vi "WriteMultipleMessages.vi"(6 "Timeout(ms)":i32, 8 "error in (no error)":errorcluster, 10 "Messages":T1[](array[typedef]), 11 "NetworkConnection in":refnum<class "NetworkConnection.lvclass">) -> (0 "error out":errorcluster, 2 "StillConnected?":bool, 3 "NetworkConnection out":refnum<class "NetworkConnection.lvclass">, 4 "Timed Out?":bool)   [LabVIEW 2020, in "NetworkConnection.lvclass"]
doc: "Writes an array of messages for the Remote System.\n\nJKI Network Streams Connection 1.1.1.15\nJavier Ruiz - JKI\nCopyright (c) 2020, JKI\n\nThis library is provided \"AS IS\" ,WITHOUT WARRANTIES OR CONDITIONS OF ANY KIND, either express or implied."
uses:
  NetworkConnection.lvclass
  NetworkCommand--Cluster.ctl
  NetworkMessage--Cluster.ctl
  NetworkConnection.lvclass/NetworkConnection.ctl
  Clear Errors.vi
  <resource>/objmgr/ni.dex.rc
panel:
  # "Copyright © 2020 JKI All rights reserved.\n\nAuthor: Javier Ruiz <javier.ruiz@jki.net>\n\nThis library is provided \"AS IS\" ,WITHOUT WARRANTIES OR \nCONDITIONS OF ANY KIND, either expressed or implied.\n\nJKI -- jki.net"
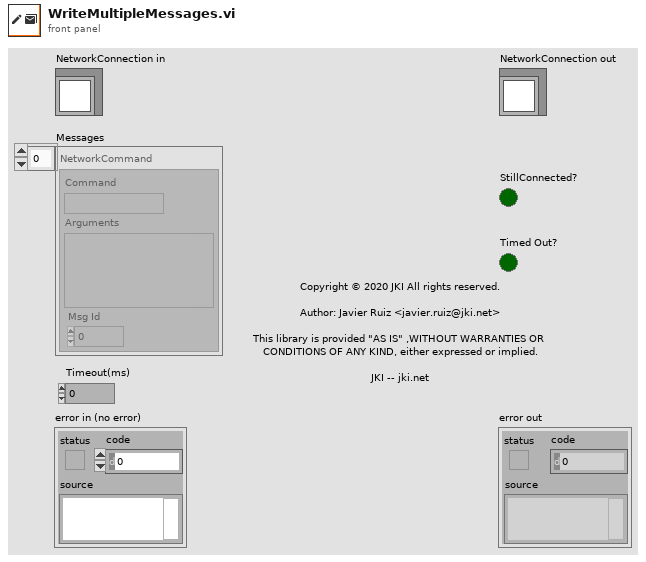
[diagram p1: front panel]
types:
  T1 = typedef "NetworkConnection.lvclass/NetworkCommand--Cluster.ctl" = cluster{"Command":string, "Arguments":variant, " Msg Id":i32}
  T2 = typedef "NetworkConnection.lvclass/NetworkMessage--Cluster.ctl" = cluster{"NetworkCommand":T1, "Wait for Ack?":bool, "Ack Id":i32}
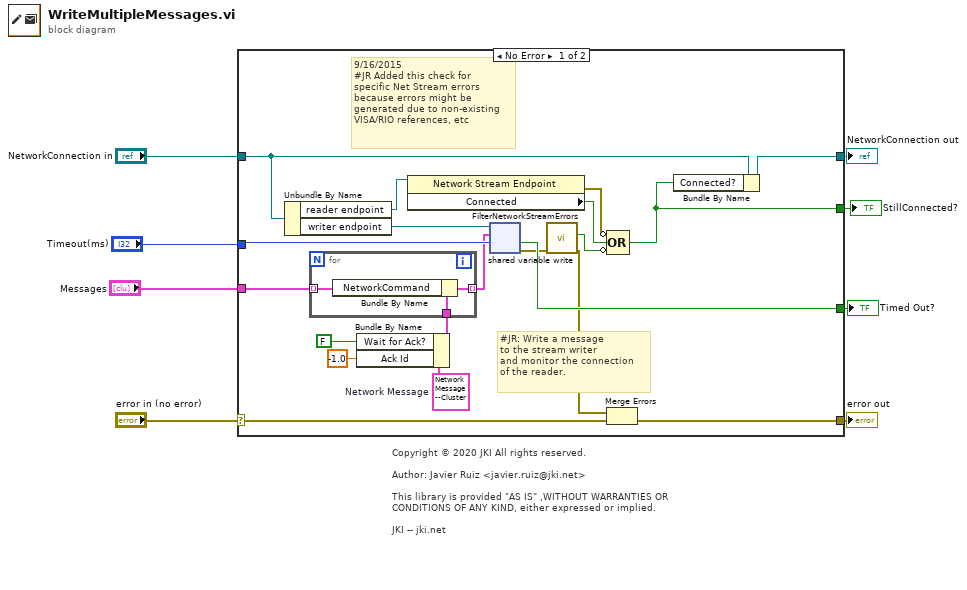
[diagram p0: block diagram]
diagram:
  # "Copyright © 2020 JKI All rights reserved.\n\nAuthor: Javier Ruiz <javier.ruiz@jki.net>\n\nThis library is provided \"AS IS\" ,WITHOUT WARRANTIES OR \nCONDITIONS OF ANY KIND, either expressed or implied.\n\nJKI -- jki.net"
  n1 = case shown="No Error" "error in (no error)" {
    selector: "error in (no error)" -> [w10 w33]
    tunnel: [w9 w33] -> w7
    tunnel: [w22 w32] -> w5
    tunnel: "NetworkConnection in" -> [w26 w32]
    tunnel: "Timeout(ms)" -> [w23 _]
    tunnel: [w21 _] -> w3
    tunnel: [w20 _] -> w2
    tunnel: "Messages" -> [w18 _]
    frame No Error {
      w24 = T2 {"NetworkCommand"={"Command"="", "Arguments"=variant, " Msg Id"=0}, "Wait for Ack?"=FALSE, "Ack Id"=0}  # Network Message
      # "9/16/2015\n#JR Added this check for\nspecific Net Stream errors\nbecause errors might be\ngenerated due to non-existing\nVISA/RIO references, etc"
      # "#JR: Write a message\nto the stream writer\nand monitor the connection\nof the reader."
      n2 = Unbundle By Name(w26) -> ("reader endpoint"=w28:refnum<k21>, "writer endpoint"=w25:refnum<k21>)
      n3 = Bundle By Name(cluster=w24, "Wait for Ack?"=FALSE ("Wait Response?"), "Ack Id"=-1.0) -> (w17:T2)
      n4 = for {
        tunnel: w18 -> [w30] mode=indexing
        tunnel: w17 -> [w31]
        tunnel: [w29] -> w16 mode=indexing
        n5 = Bundle By Name(cluster=w31, "NetworkCommand"=w30) -> (w29:T2)
      }
      n6 = property class="Network Stream Endpoint"(reference=w28) -> (error out=w14:errorcluster, "Connected"=w27:bool)  [unwired: 1 in, 1 out]
      n7 = shared-variable-write(w25, w16, w23) -> (w13:errorcluster, w20:bool)  [unwired: 1 in, 1 out]
      n8 = call "FilterNetworkStreamErrors.vi"("error in (no error)"=w13) -> ("error out"=w11:errorcluster, "NetStream Error?"=w12:bool)  [unwired: 9 in]
      n9 = Compound Arithmetic op=OR(invert w14, w27, invert w12) -> (w21:bool)
      n10 = Merge Errors(w11, w10) -> (w9:errorcluster)
      n11 = Bundle By Name(cluster=w26, "Connected?"=w21) -> (w22:refnum<class "NetworkConnection.lvclass">)
    }
    frame Error {
    }
  }
  "error out" <- w7
  "NetworkConnection out" <- w5
  "StillConnected?" <- w3
  "Timed Out?" <- w2
